vi "scan_laser_to_value.vi"(6 "Error range":dbl, 7 "address":string, 8 "error in":errorcluster, 9 "Scan Speed":dbl, 10 "Target Value":dbl, 11 "Measure Type":enum16{"Wavelength", "Wavenumber"}(ring)) -> (0 "error out":errorcluster, 2 "Finished Move?":bool)   [LabVIEW 2020]
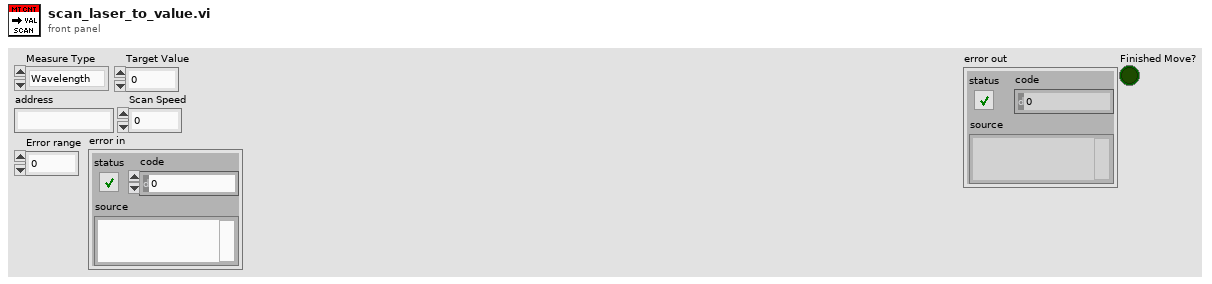
[diagram p1: front panel]
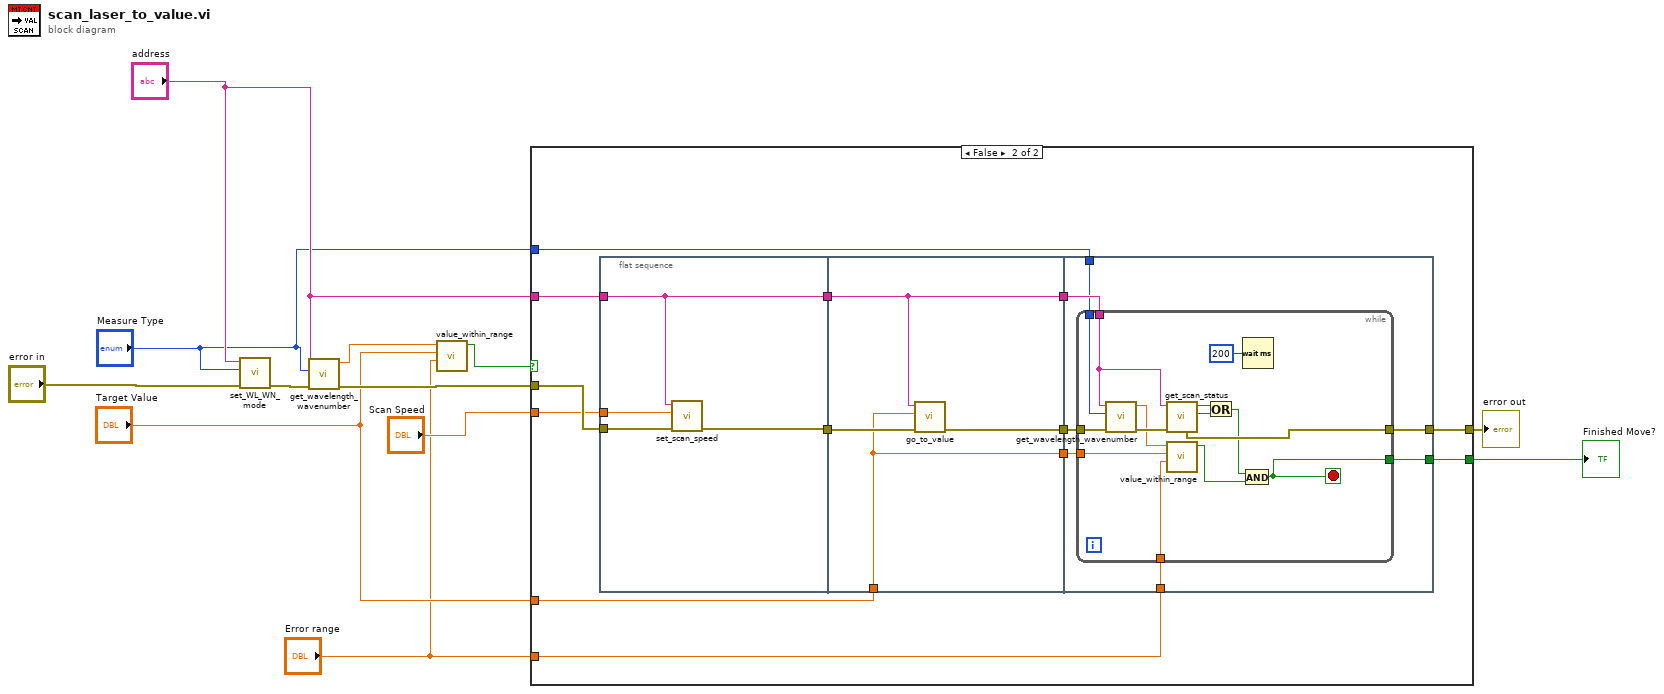
[diagram p0: block diagram]
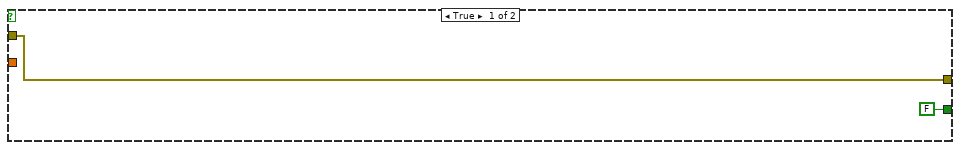
[diagram p2: hidden frame]
diagram:
  n1 = call "set_WL_WN_mode.vi"("error in"="error in", "Measure Type"="Measure Type", "address"="address") -> ("error out"=w12:errorcluster)  [unwired: 8 in]
  n2 = call "get_wavelength_wavenumber.vi"("error in"=w12, "Measure Type"="Measure Type", "address"="address") -> ("error out"=w10:errorcluster, "Wavelength/Wavenuumber"=w4:dbl)  [unwired: 7 in]
  n3 = call "value_within_range.vi"("Error range"="Error range", "Target Value"="Target Value", "Actual Value"=w4) -> ("within_range?"=w1:bool)  [unwired: 8 in]
  n4 = case shown="False" w1 {
    tunnel: "address" -> [_ w27]
    tunnel: w10 -> [w14 w26]
    tunnel: "Scan Speed" -> [_ w24]
    tunnel: "Target Value" -> [_ w21]
    tunnel: "Measure Type" -> [_ w19]
    tunnel: "Error range" -> [_ w17]
    tunnel: [w14 w15] -> w6
    tunnel: [FALSE w16] -> w5
    frame True {
    }
    frame False {
      n5 = flat-sequence {
        tunnel: w27 -> [w28]
        tunnel: w26 -> [w31]
        tunnel: [w30] -> w25
        tunnel: w24 -> [w29]
        tunnel: [w28] -> w22
        tunnel: w25 -> [w35]
        tunnel: [w34] -> w23
        tunnel: w22 -> [w33]
        tunnel: w21 -> [w32]
        tunnel: [w33] -> w20
        tunnel: [w32] -> w18
        tunnel: w23 -> [w42]
        tunnel: w20 -> [w41]
        tunnel: w19 -> [w40]
        tunnel: w18 -> [w39]
        tunnel: w17 -> [w38]
        tunnel: [w37] -> w15
        tunnel: [w36] -> w16
        frame #0 {
          n6 = call "set_scan_speed.vi"("error in"=w31, "Scan Speed"=w29, "address"=w28) -> ("error out"=w30:errorcluster)  [unwired: 8 in]
        }
        frame #1 {
          n7 = call "go_to_value.vi"("error in"=w35, "Target Value"=w32, "address"=w33) -> ("error out"=w34:errorcluster)  [unwired: 8 in]
        }
        frame #2 {
          n8 = while {
            tunnel: w42 -> [w56]
            tunnel: w41 -> [w54]
            tunnel: w40 -> [w53]
            tunnel: w39 -> [w51]
            tunnel: w38 -> [w50]
            tunnel: [w48] -> w37
            tunnel: [w46] -> w36
            stop <- w46 stop-if-true
            n9 = call "get_wavelength_wavenumber.vi"("error in"=w56, "Measure Type"=w53, "address"=w54) -> ("error out"=w55:errorcluster, "Wavelength/Wavenuumber"=w52:dbl)  [unwired: 7 in]
            n10 = call "get_scan_status.vi"("error in"=w55, "address"=w54) -> ("Reducing Errors?"=w44:bool, "Scan Finished?"=w45:bool, "error out"=w48:errorcluster)  [unwired: 5 in, 2 out]
            n11 = call "value_within_range.vi"("Error range"=w50, "Target Value"=w51, "Actual Value"=w52) -> ("within_range?"=w49:bool)  [unwired: 8 in]
            n12 = Or(x=w45, y=w44) -> (x .or. y?=w43:bool)
            n13 = And(x=w43, y=w49) -> (x .and. y?=w46:bool)
            n14 = Wait (ms)(milliseconds to wait=u32 200) -> ()  [unwired: 1 out]
          }
        }
      }
    }
  }
  "error out" <- w6
  "Finished Move?" <- w5
